vi "subDFD_Remez Design Example Data.vi"(0 "Example Idx":i32=13) -> (1 "minimum order":enum32{"User Defined", "MinEven", "MinOdd"}(ring), 2 "description":string="Designs an arbitrary shape lowpass filter. The passband response is an anti-sinc function x/sin(x).", 3 "phase option":T2, 4 "order":i32=50, 5 "band specs":T1[](array[typedef])=[{"band specification"=array[5000 elements], "ripple constraint"=0.0}, {"band specification"=[{"freq"=0.3, "amplitude"=0.0, "weight"=1.0}, {"freq"=0.5, "amplitude"=0.0, "weight"=1.0}], "ripple constraint"=0.0}], 6 "freqs of exact gain":dbl[](array[numeric]))   [LabVIEW 2023]
uses:
  <vilib>/addons/Digital Filter Design/_REMEZ.llb/remez_fir filter type.ctl
  <vilib>/addons/Digital Filter Design/_Objects.llb/DFD Adv Band Spec.ctl
  <vilib>/addons/Digital Filter Design/NI_DigFilterLicensed.lvlib
panel:
  in  "Example Descriptions":string[](array[string])=["Designs a lowpass filter with a higher weight in the stopband than in the passband. The resulting filter has a smaller stopband ripple than passband ripple. The default weighting values of the passband and stopband of this example are 1 and 5, respectively. The resulting passband ripple size is 5 times the stopband ripple size. Switch to the Specifications page to examine the filter specifications for this example.", "Designs a lowpass filter with a higher weight in the passband than in the stopband. The resulting filter has a smaller passband ripple than stopband ripple. The default weighting values of the passband and stopband of this example are 5 and 1, respectively. The resulting passband ripple size is one-fifth the stopband ripple size. Switch to the Specifications page to examine the filter specifications for this example.", "Designs an antisymmetric highpass filter. Only odd order is allowed in this filter. ", "Designs a ripple-shaped bandpass filter that allows variable inband weighting values. This example demonstrates a Least Square alike bandpass filter design by specifying variable inband weighting values for each band.", "Designs a bandstop filter with the stopband constrained to be less than 0.1 and the passband not constrained. To achieve the minimal passband ripple size, the algorithm adjusts the stopband value within its constraint for the fixed filter order.", "Designs a bandstop filter that has two constrained passbands with different constraint values, 0.05 and 0.1, and the stopband is not constrained. To achieve the minimal stopband ripple size, the algorithm adjusts the passband values within their respective constraints for the fixed filter order. ", "Designs a single-point band filter that has two single-point bands that are also specified in Frequencies of Exact Gain. At frequencies 0.125 and 0.275, the frequency response of this filter passes at exactly zero.", "Designs a highpass filter with exact gain control at 0.015. To view the zero-crossing at the specified frequency, zoom in on the magnitude response of the designed filter. You can change this frequency value or add more values to the Frequencies of Exact Gain array on the Specifications page. Click the Apply button on the Specifications page to see how the magnitude response changes when you redesign the filter.", "Designs a lowpass filter with the constrained passband and stopband ripples specified as 0.1 and 0.02 respectively. The DFD Remez Design VI designs a minimum even-order filter to satisfy the constraints.", "Designs a lowpass filter with the stopband ripple constrained to be less than 0.1. This is a minimum phase design by default. The phase response of the filter is not linear.\nBy changing the Filter Type to Symmetric and redesigning the filter, you can see the difference between linear phase and minimum phase filters with the same order. The minimum phase filter has a smaller ripple size.\n", "Designs an optimal minimum phase multiband filter with different stopband ripple sizes.", "Designs an even-order differentiator.", "Designs an even-order Hilbert transformer.", "Designs an arbitrary shape lowpass filter. The passband response is an anti-sinc function x/sin(x)."]
  in  "Example Settings":T3(array[cluster])=[{"order"=22, "phase option"=enum."Symmetric", "minimum order"=enum."User Defined", "band specs"=[{"band specification"=[{"freq"=0.0, "amplitude"=1.0, "weight"=1.0}, {"freq"=0.2, "amplitude"=1.0, "weight"=1.0}], "ripple constraint"=0.0}, {"band specification"=[{"freq"=0.25, "amplitude"=0.0, "weight"=5.0}, {"freq"=0.5, "amplitude"=0.0, "weight"=5.0}], "ripple constraint"=0.0}]}, {"order"=22, "phase option"=enum."Symmetric", "minimum order"=enum."User Defined", "band specs"=[{"band specification"=[{"freq"=0.0, "amplitude"=1.0, "weight"=5.0}, {"freq"=0.2, "amplitude"=1.0, "weight"=5.0}], "ripple constraint"=0.0}, {"band specification"=[{"freq"=0.25, "amplitude"=0.0, "weight"=1.0}, {"freq"=0.5, "amplitude"=0.0, "weight"=1.0}], "ripple constraint"=0.0}]}, {"order"=21, "phase option"=enum."Antisymmetric", "minimum order"=enum."User Defined", "band specs"=[{"band specification"=[{"freq"=0.0, "amplitude"=0.0, "weight"=2.0}, {"freq"=0.2, "amplitude"=0.0, "weight"=2.0}], "ripple constraint"=0.0}, {"band specification"=[{"freq"=0.25, "amplitude"=1.0, "weight"=1.0}, {"freq"=0.5, "amplitude"=1.0, "weight"=1.0}], "ripple constraint"=0.0}]}, {"order"=53, "phase option"=enum."Symmetric", "minimum order"=enum."User Defined", "band specs"=[{"band specification"=[{"freq"=0.0, "amplitude"=0.0, "weight"=5.0}, {"freq"=0.03, "amplitude"=0.0, "weight"=4.618033988749895}, {"freq"=0.06, "amplitude"=0.0, "weight"=3.618033988749895}, {"freq"=0.09, "amplitude"=0.0, "weight"=2.381966011250105}, {"freq"=0.12, "amplitude"=0.0, "weight"=1.3819660112501053}, {"freq"=0.15, "amplitude"=0.0, "weight"=1.0}], "ripple constraint"=0.0}, {"band specification"=[{"freq"=0.165, "amplitude"=1.0, "weight"=1.0}, {"freq"=0.185, "amplitude"=1.0, "weight"=1.3174929343376376}, {"freq"=0.205, "amplitude"=1.0, "weight"=2.169169973996227}, {"freq"=0.22499999999999998, "amplitude"=1.0, "weight"=3.28462967654657}, {"freq"=0.24499999999999997, "amplitude"=1.0, "weight"=4.30972146789057}, {"freq"=0.26499999999999996, "amplitude"=1.0, "weight"=4.918985947228995}, {"freq"=0.285, "amplitude"=1.0, "weight"=4.918985947228995}, {"freq"=0.305, "amplitude"=1.0, "weight"=4.30972146789057}, {"freq"=0.325, "amplitude"=1.0, "weight"=3.2846296765465706}, {"freq"=0.34500000000000003, "amplitude"=1.0, "weight"=2.169169973996228}, {"freq"=0.36500000000000005, "amplitude"=1.0, "weight"=1.3174929343376376}, {"freq"=0.38500000000000006, "amplitude"=1.0, "weight"=1.0}], "ripple constraint"=0.0}, {"band specification"=[{"freq"=0.4, "amplitude"=0.0, "weight"=0.5}, {"freq"=0.42000000000000004, "amplitude"=0.0, "weight"=0.6909830056250524}, {"freq"=0.44000000000000006, "amplitude"=0.0, "weight"=1.1909830056250525}, {"freq"=0.4600000000000001, "amplitude"=0.0, "weight"=1.8090169943749472}, {"freq"=0.4800000000000001, "amplitude"=0.0, "weight"=2.3090169943749475}, {"freq"=0.5, "amplitude"=0.0, "weight"=2.5}], "ripple constraint"=0.0}]}, {"order"=12, "phase option"=enum."Symmetric", "minimum order"=enum."User Defined", "band specs"=[{"band specification"=[{"freq"=0.0, "amplitude"=1.0, "weight"=1.0}, {"freq"=0.2, "amplitude"=1.0, "weight"=1.0}], "ripple constraint"=0.0}, {"band specification"=[{"freq"=0.25, "amplitude"=0.0, "weight"=1.0}, {"freq"=0.5, "amplitude"=0.0, "weight"=1.0}], "ripple constraint"=0.1}]}, {"order"=22, "phase option"=enum."Symmetric", "minimum order"=enum."User Defined", "band specs"=[{"band specification"=[{"freq"=0.0, "amplitude"=1.0, "weight"=1.0}, {"freq"=0.2, "amplitude"=1.0, "weight"=1.0}], "ripple constraint"=0.05}, {"band specification"=[{"freq"=0.25, "amplitude"=0.0, "weight"=1.0}, {"freq"=0.35, "amplitude"=0.0, "weight"=1.0}], "ripple constraint"=0.0}, {"band specification"=[{"freq"=0.4, "amplitude"=1.0, "weight"=1.0}, {"freq"=0.5, "amplitude"=1.0, "weight"=1.0}], "ripple constraint"=0.1}]}, {"order"=42, "phase option"=enum."Symmetric", "minimum order"=enum."User Defined", "band specs"=[{"band specification"=[{"freq"=0.0, "amplitude"=1.0, "weight"=1.0}, {"freq"=0.1, "amplitude"=1.0, "weight"=1.0}], "ripple constraint"=0.0}, {"band specification"=[{"freq"=0.125, "amplitude"=0.0, "weight"=10.0}], "ripple constraint"=0.0}, {"band specification"=[{"freq"=0.15, "amplitude"=1.0, "weight"=1.0}, {"freq"=0.25, "amplitude"=1.0, "weight"=1.0}], "ripple constraint"=0.0}, {"band specification"=[{"freq"=0.275, "amplitude"=0.0, "weight"=10.0}], "ripple constraint"=0.0}, {"band specification"=[{"freq"=0.3, "amplitude"=1.0, "weight"=1.0}, {"freq"=0.5, "amplitude"=1.0, "weight"=1.0}], "ripple constraint"=0.0}]}, {"order"=82, "phase option"=enum."Symmetric", "minimum order"=enum."User Defined", "band specs"=[{"band specification"=[{"freq"=0.0, "amplitude"=0.0, "weight"=1.0}, {"freq"=0.00275, "amplitude"=0.0, "weight"=1.0}, {"freq"=0.015, "amplitude"=0.0, "weight"=1.0}, {"freq"=0.05, "amplitude"=0.0, "weight"=1.0}], "ripple constraint"=0.0}, {"band specification"=[{"freq"=0.075, "amplitude"=1.0, "weight"=1.0}, {"freq"=0.5, "amplitude"=1.0, "weight"=1.0}], "ripple constraint"=0.0}]}, {"order"=0, "phase option"=enum."Symmetric", "minimum order"=enum."MinEven", "band specs"=[{"band specification"=[{"freq"=0.0, "amplitude"=1.0, "weight"=1.0}, {"freq"=0.2, "amplitude"=1.0, "weight"=1.0}], "ripple constraint"=0.1}, {"band specification"=[{"freq"=0.25, "amplitude"=0.0, "weight"=1.0}, {"freq"=0.5, "amplitude"=0.0, "weight"=1.0}], "ripple constraint"=0.02}]}, {"order"=12, "phase option"=enum."Minimum Phase", "minimum order"=enum."User Defined", "band specs"=[{"band specification"=[{"freq"=0.0, "amplitude"=1.0, "weight"=1.0}, {"freq"=0.2, "amplitude"=1.0, "weight"=1.0}], "ripple constraint"=0.0}, {"band specification"=[{"freq"=0.25, "amplitude"=0.0, "weight"=1.0}, {"freq"=0.5, "amplitude"=0.0, "weight"=1.0}], "ripple constraint"=0.1}]}, {"order"=24, "phase option"=enum."Minimum Phase", "minimum order"=enum."User Defined", "band specs"=[{"band specification"=[{"freq"=0.0, "amplitude"=0.0, "weight"=1.0}, {"freq"=0.13, "amplitude"=0.0, "weight"=1.0}], "ripple constraint"=0.0}, {"band specification"=[{"freq"=0.15, "amplitude"=1.0, "weight"=1.0}, {"freq"=0.3, "amplitude"=1.0, "weight"=1.0}], "ripple constraint"=0.0}, {"band specification"=[{"freq"=0.32, "amplitude"=0.0, "weight"=2.0}, {"freq"=0.5, "amplitude"=0.0, "weight"=2.0}], "ripple constraint"=0.0}]}, {"order"=20, "phase option"=enum."Differentiator", "minimum order"=enum."User Defined", "band specs"=[{"band specification"=[{"freq"=0.1, "amplitude"=0.1, "weight"=1.0}, {"freq"=0.4, "amplitude"=0.4, "weight"=1.0}], "ripple constraint"=0.0}]}, {"order"=20, "phase option"=enum."Hilbert", "minimum order"=enum."MinEven", "band specs"=[{"band specification"=[{"freq"=0.02, "amplitude"=1.0, "weight"=1.0}, {"freq"=0.45, "amplitude"=1.0, "weight"=1.0}], "ripple constraint"=0.1}]}, {"order"=50, "phase option"=enum."Symmetric", "minimum order"=enum."User Defined", "band specs"=[{"band specification"=array[5000 elements], "ripple constraint"=0.0}, {"band specification"=[{"freq"=0.3, "amplitude"=0.0, "weight"=1.0}, {"freq"=0.5, "amplitude"=0.0, "weight"=1.0}], "ripple constraint"=0.0}]}]
  # "freq"
  # "amplitude"
  # "weight"
  # "freq"
  # "amplitude"
  # "weight"
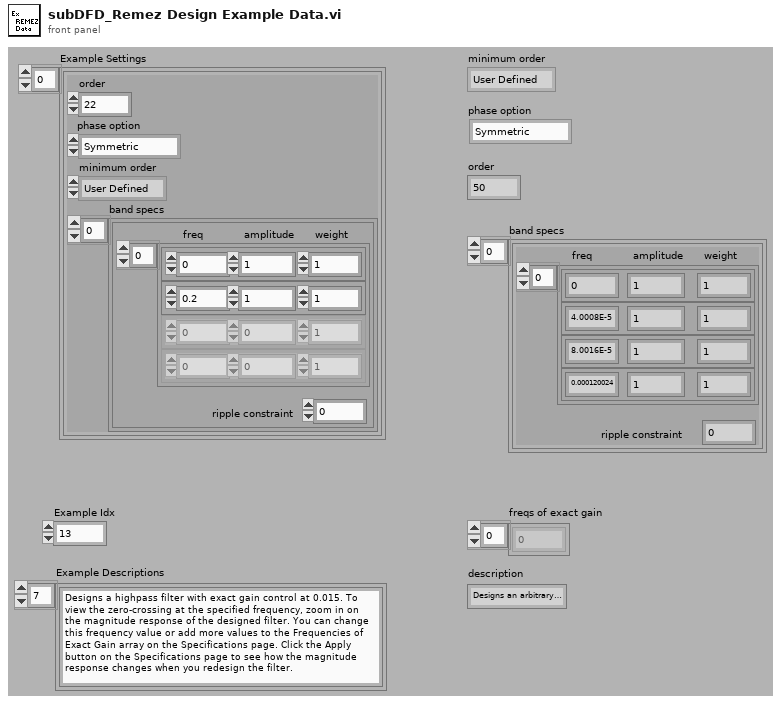
[diagram p1: front panel]
types:
  T1 = typedef "NI_DigFilterLicensed.lvlib/DFD Adv Band Spec.ctl" = cluster{"band specification":cluster{"freq":dbl, "amplitude":dbl, "weight":dbl}[], "ripple constraint":dbl}
  T2 = typedef "NI_DigFilterLicensed.lvlib/remez_fir filter type.ctl" = enum32{"Symmetric", "Antisymmetric", "Differentiator", "Hilbert", "Minimum Phase", "Maximum Phase"}
  T3 = cluster{"order":i32, "phase option":T2, "minimum order":enum32{"User Defined", "MinEven", "MinOdd"}, "band specs":T1[]}[]
  T4 = cluster{"order":i32, "phase option":T2, "minimum order":enum32{"User Defined", "MinEven", "MinOdd"}, "band specs":T1[]}
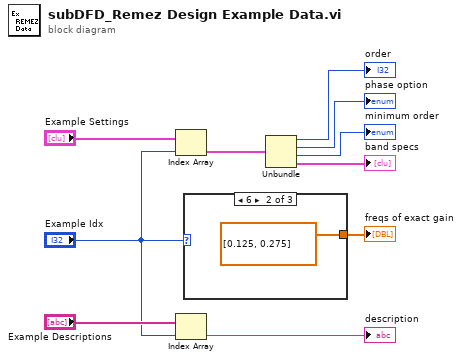
[diagram p0: block diagram]
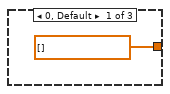
[diagram p2: hidden frame]
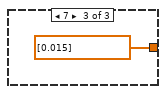
[diagram p3: hidden frame]
diagram:
  n1 = Index Array(array="Example Settings", index="Example Idx") -> (element=w9:T4)
  n2 = Index Array(array="Example Descriptions", index="Example Idx") -> (element=→"description":string)
  n3 = case shown="6" "Example Idx" {
    tunnel: [dbl[] [] dbl[] [0.125, 0.275] dbl[] [0.015]] -> w4
    frame 0, Default {
    }
    frame 6 {
    }
    frame 7 {
    }
  }
  "freqs of exact gain" <- w4
  n4 = Unbundle(w9) -> ("order"=→"order":i32, "phase option"=→"phase option":T2, "minimum order"=→"minimum order":enum32{"User Defined", "MinEven", "MinOdd"}, "band specs"=→"band specs":T1[])
